vi "BROOKFIELD_EXT-MODE_STATE.vi"() -> ()   [LabVIEW 2019]
uses:
  Brookfield_type-def.ctl
  <vilib>/Instr/_visa.llb/VISA Configure Serial Port (Instr).vi
panel:
  out "error out":errorcluster
  in  "Conductivity Port":refnum<visa-resource-name>="COM5"
  in  "Read Stop":bool
  in  "Disconnect":bool
  out "Enum":T1
  in  "Read Start":bool
  in  "Stop":bool
  in  "Set Speed":bool
  in  "Zero":bool
  out "temp":dbl
  out "torque%":dbl
  out "Control Circuitry Enabled":bool
  out "Motor On":bool
  out "Motor Stopped":bool
  out "Auto-zero Complete":bool
  out "Motor Circuit Error":bool
  out "Diagnostics Error":bool
  out "Invalid Command Received":bool
  out "Torque% Offset":dbl
  in  "rpm setpoint":i32=60
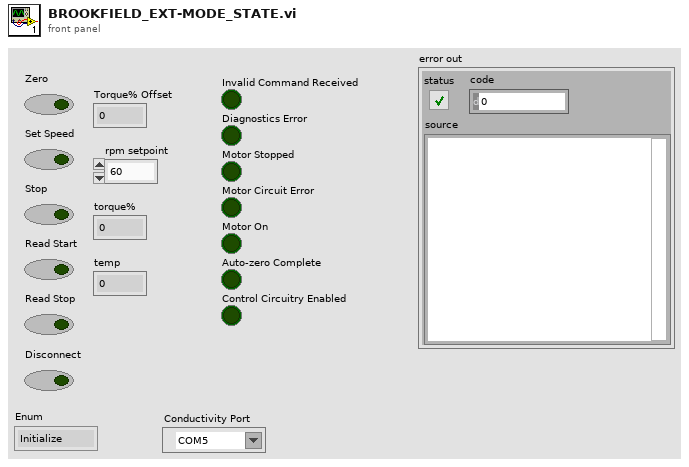
[diagram p1: front panel]
types:
  T1 = typedef "Brookfield_type-def.ctl" = enum16{"Initialize", "Enable", "Ready", "Zero", "Set Speed", "Read", "Stop Motor", "Error", "Disconnect"}
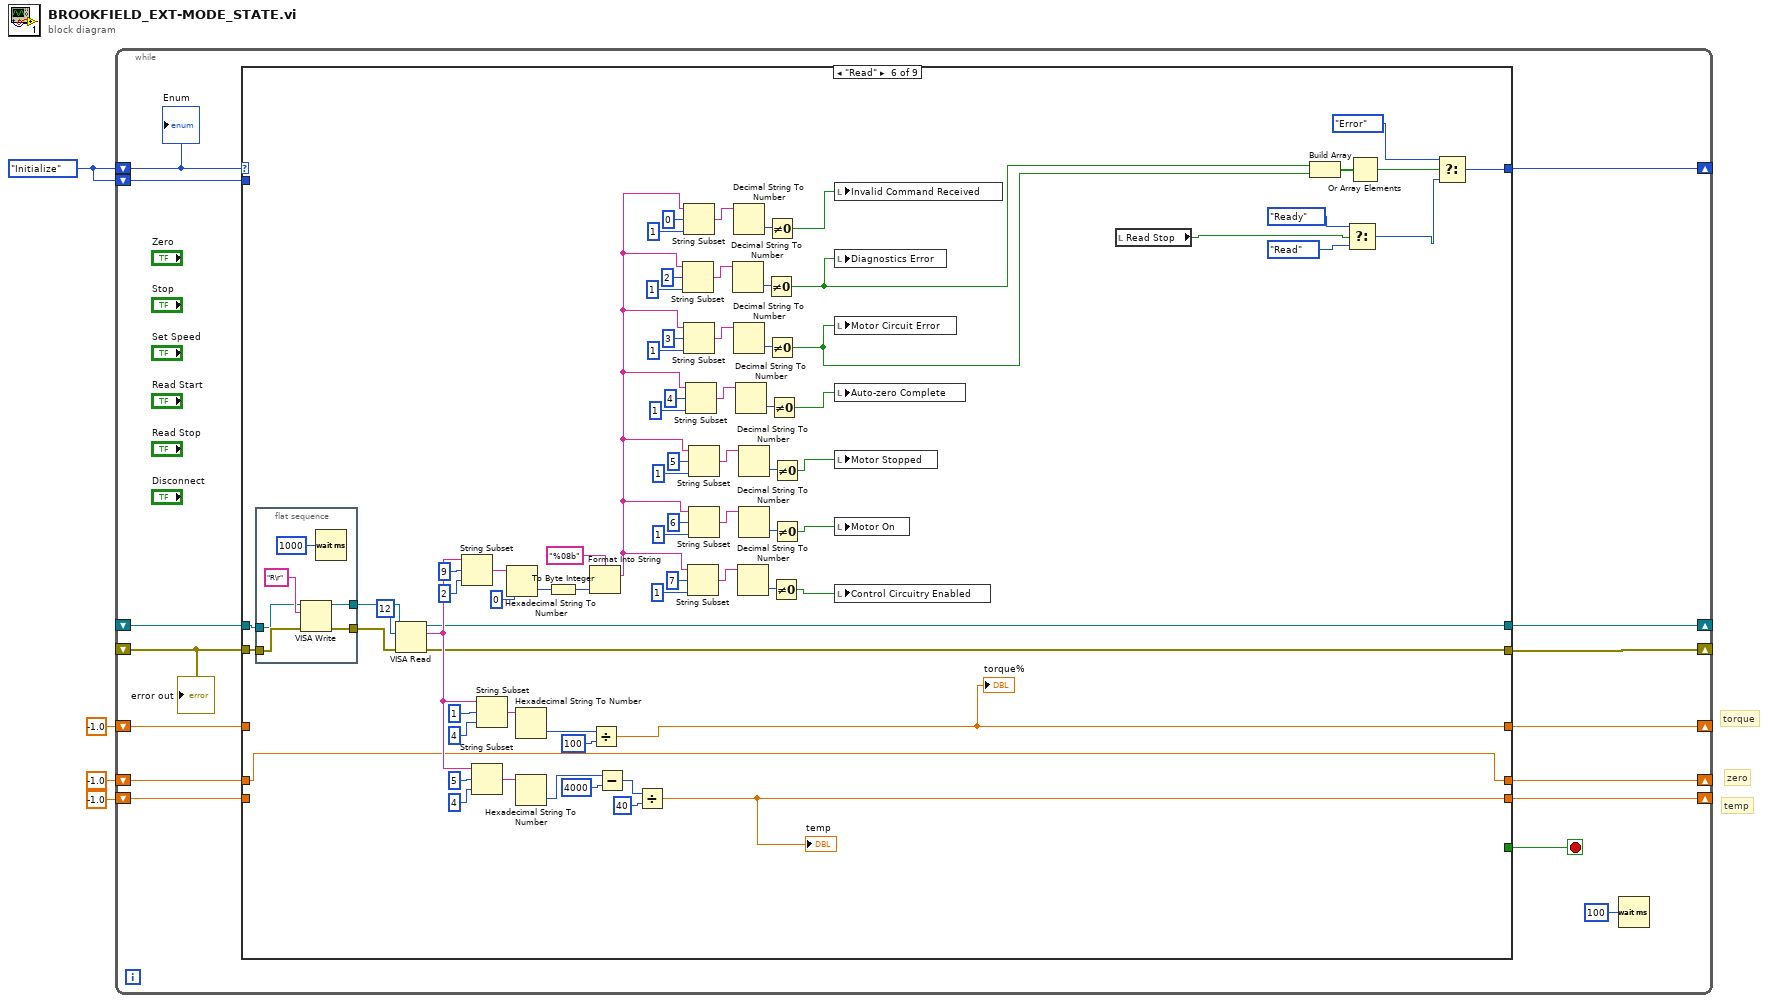
[diagram p0: block diagram]
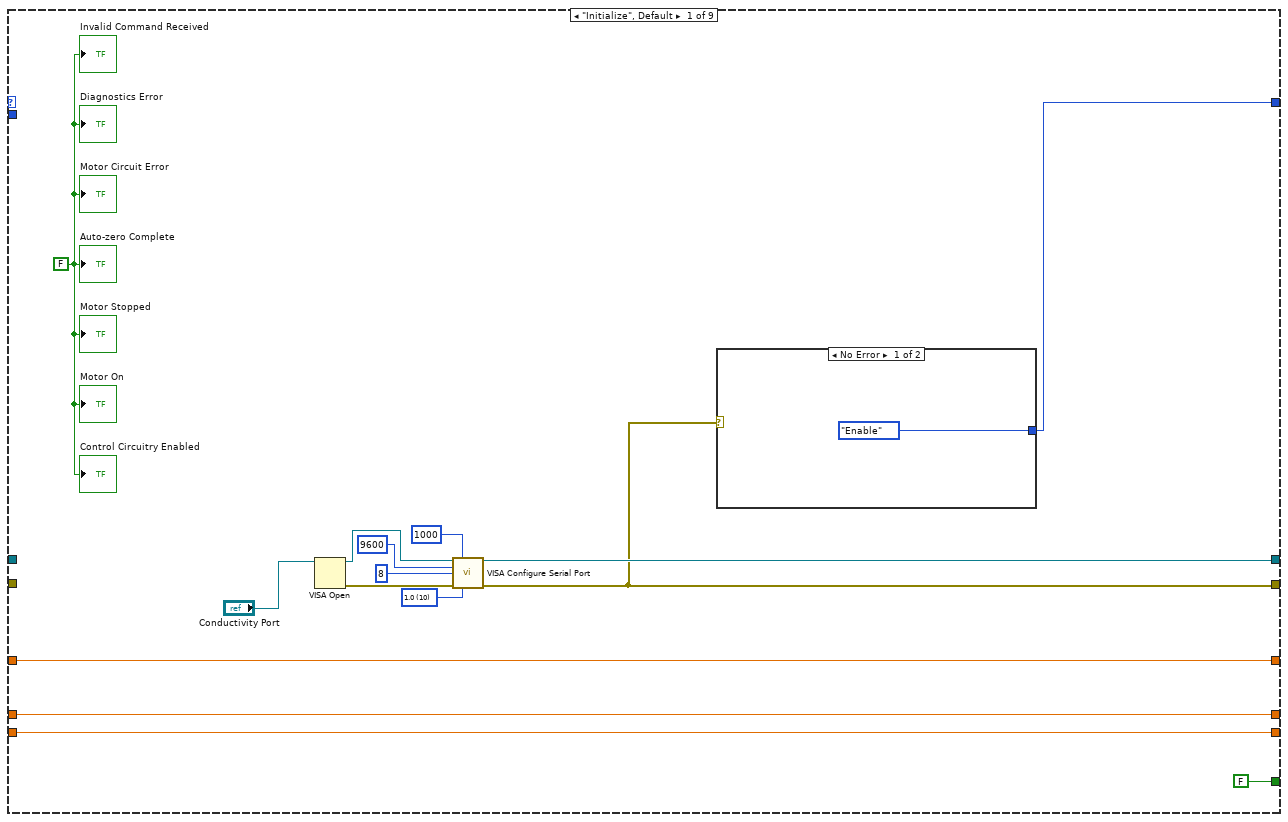
[diagram p2: hidden frame]
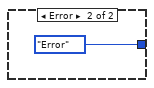
[diagram p3: hidden frame]
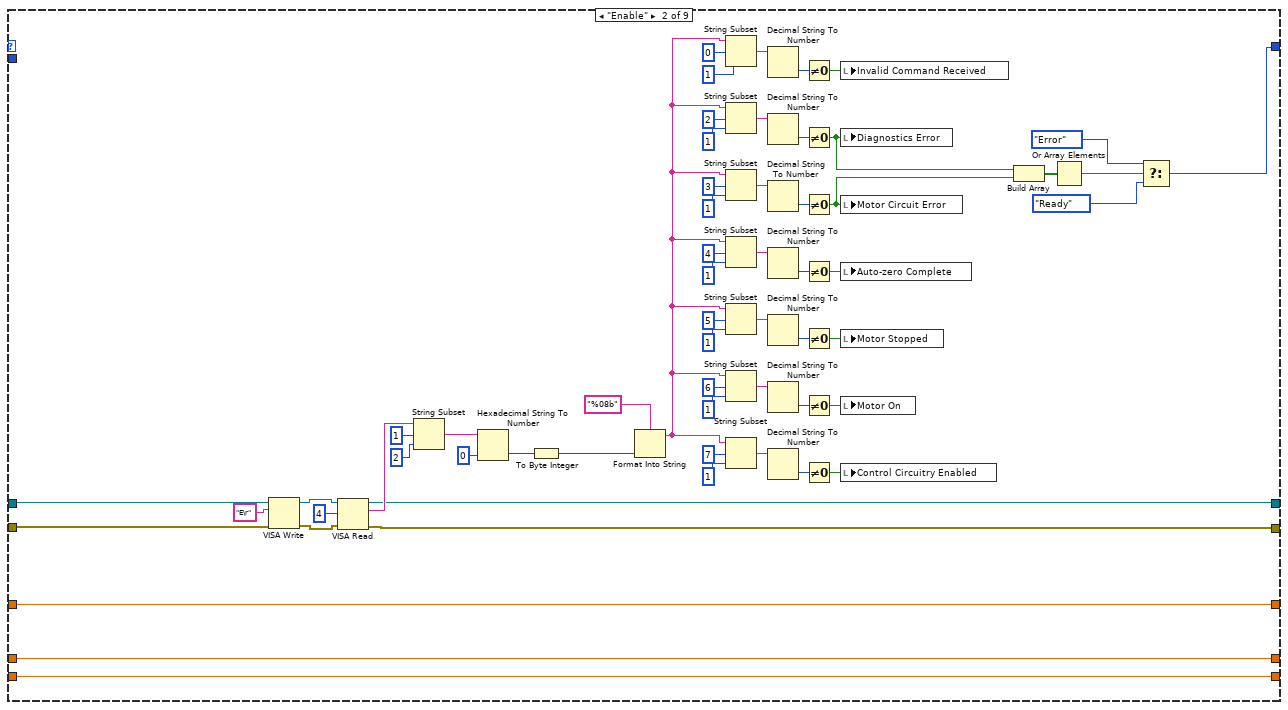
[diagram p4: hidden frame]
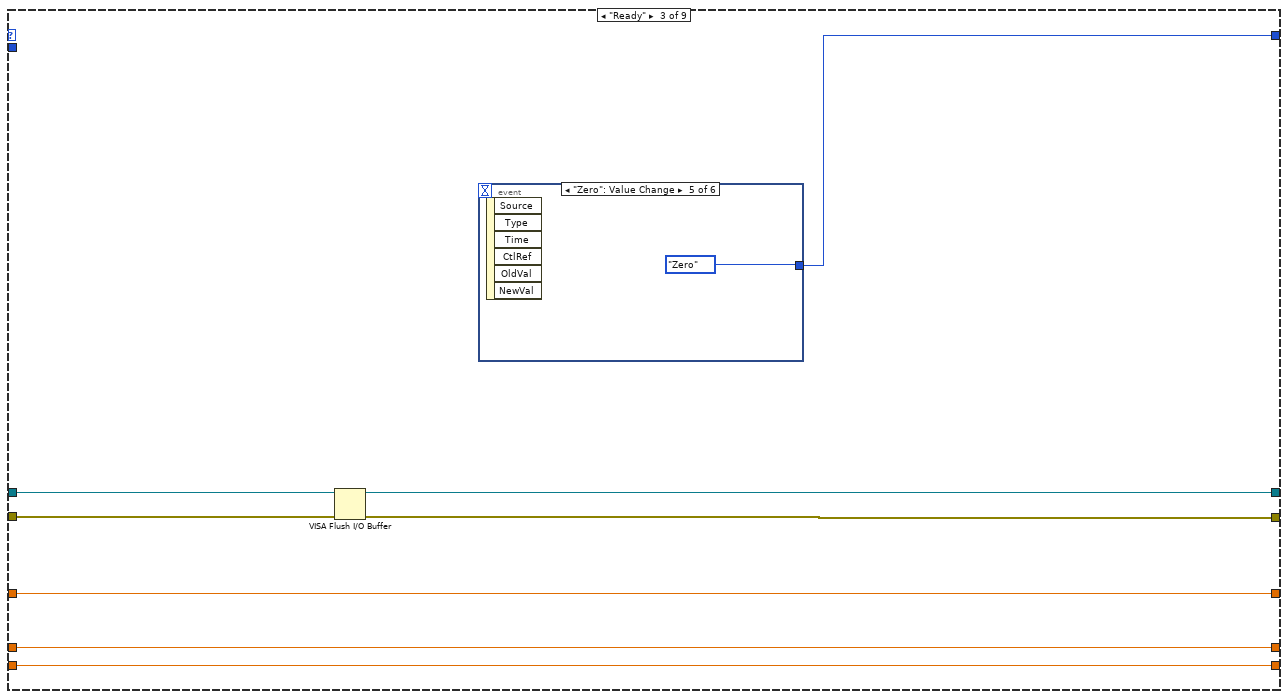
[diagram p5: hidden frame]
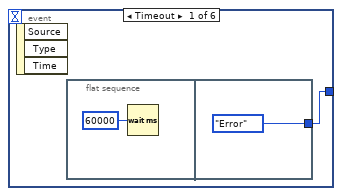
[diagram p6: hidden frame]
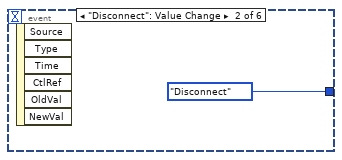
[diagram p7: hidden frame]
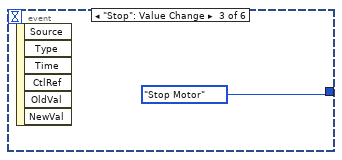
[diagram p8: hidden frame]
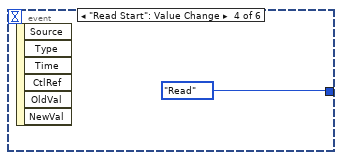
[diagram p9: hidden frame]
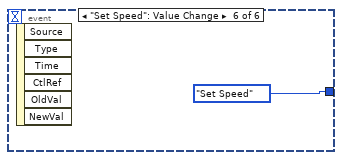
[diagram p10: hidden frame]
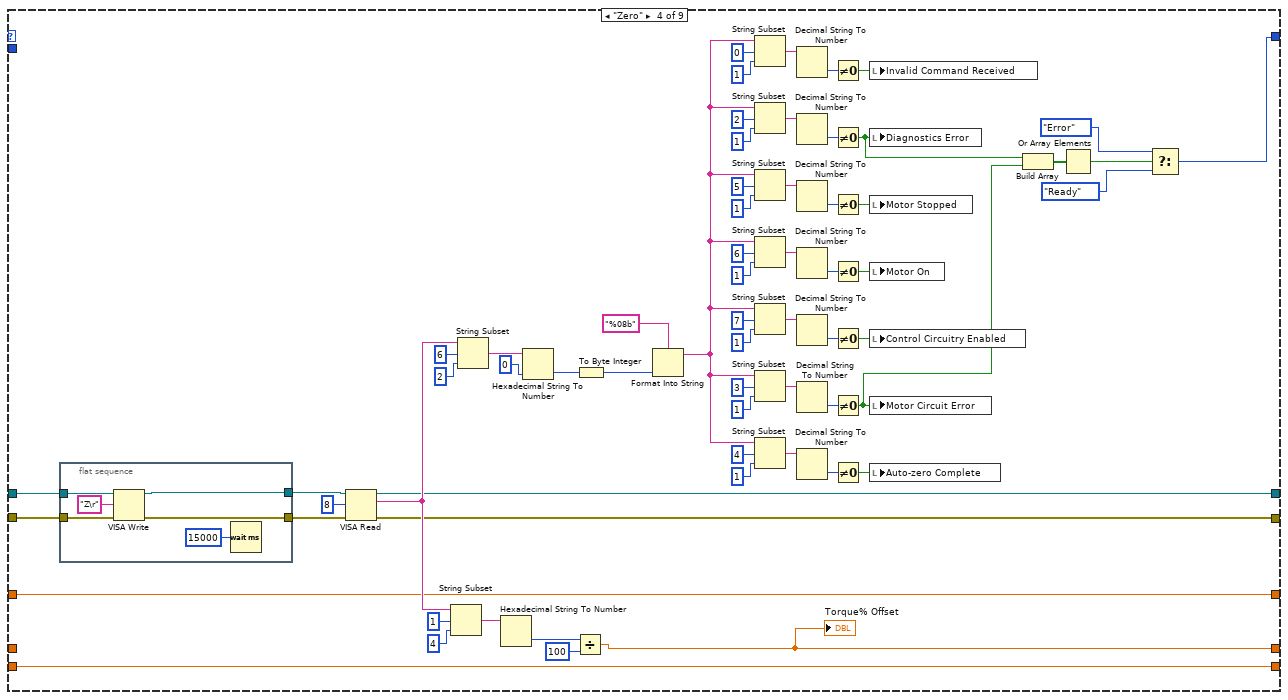
[diagram p11: hidden frame]
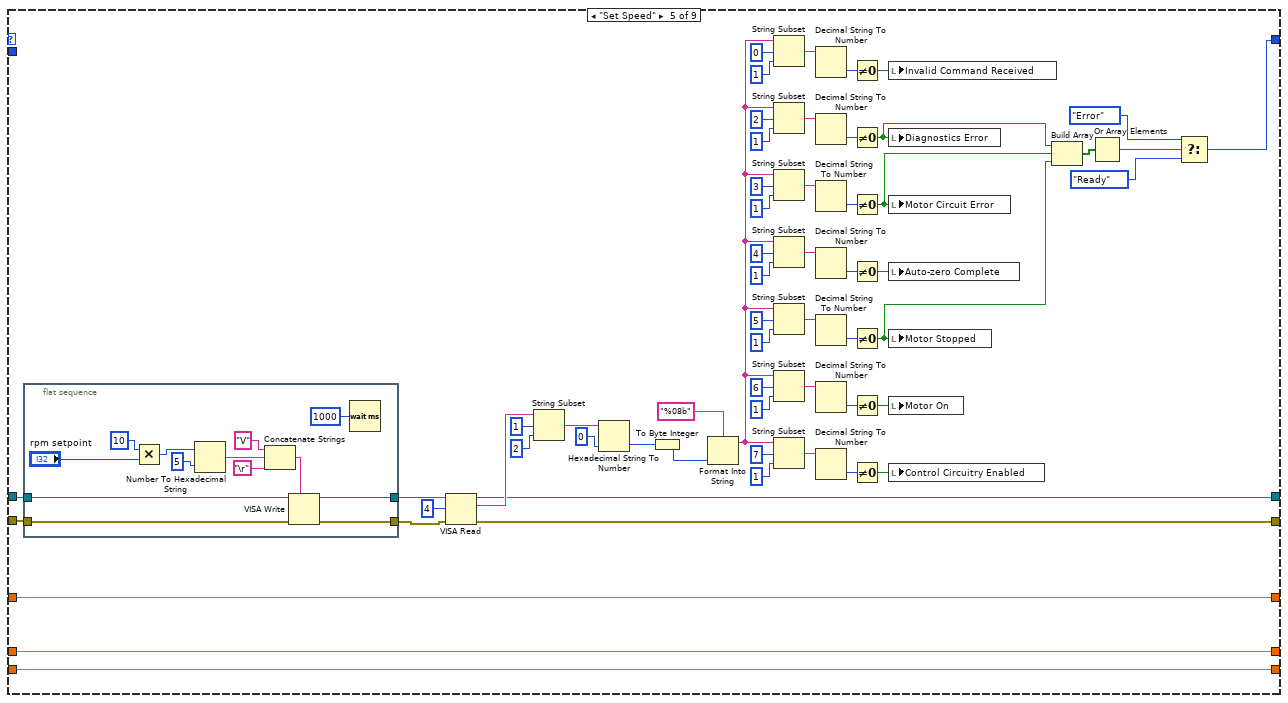
[diagram p12: hidden frame]
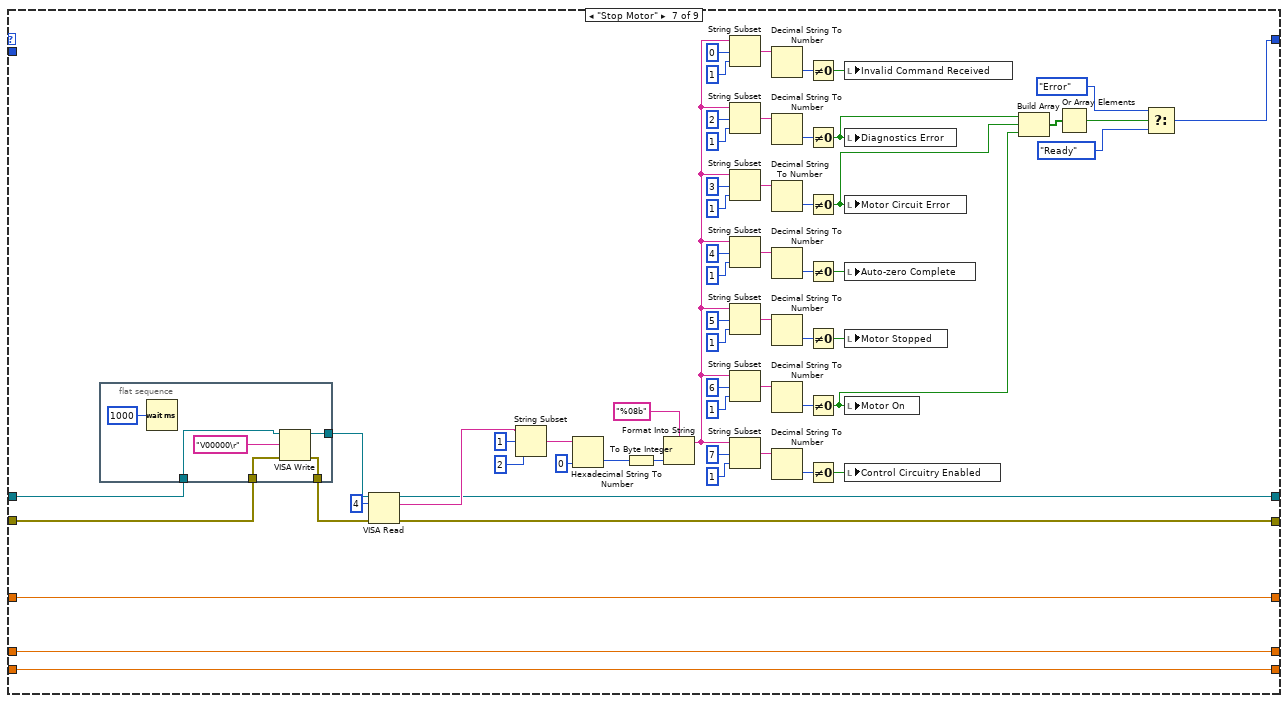
[diagram p13: hidden frame]
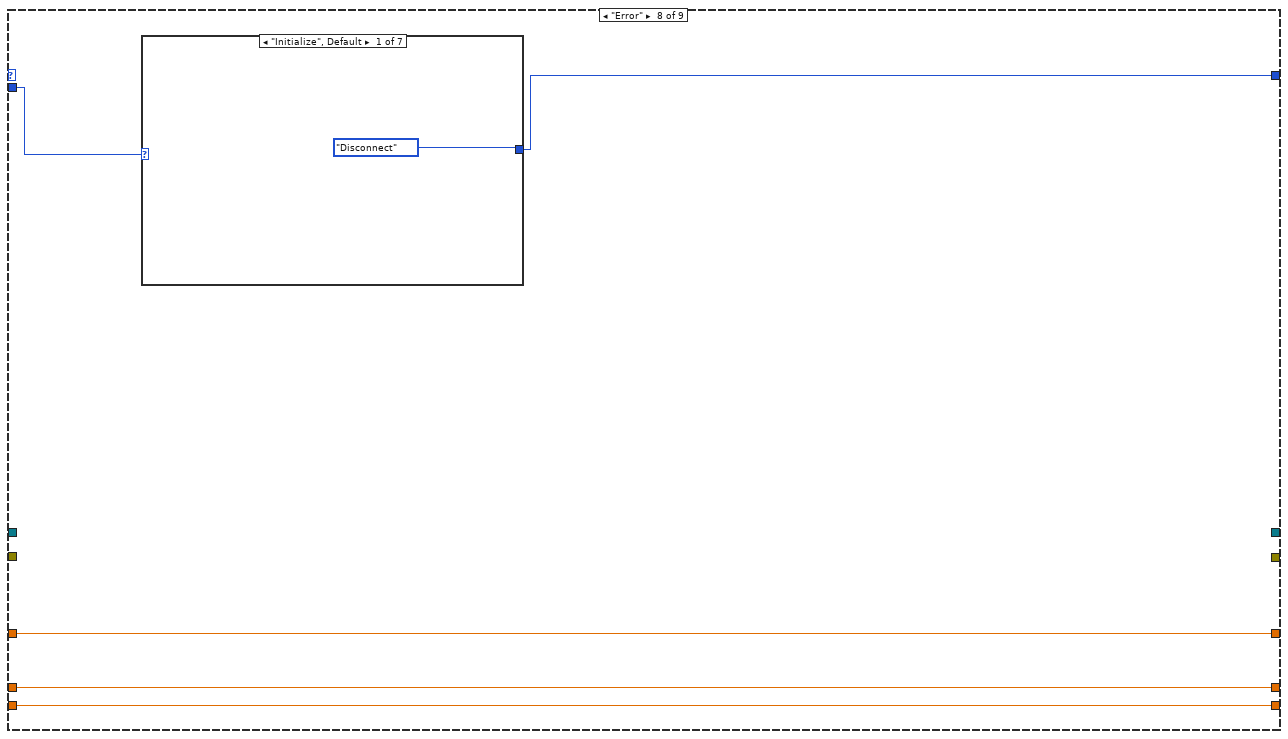
[diagram p14: hidden frame]
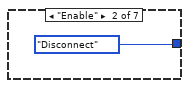
[diagram p15: hidden frame]
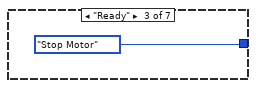
[diagram p16: hidden frame]
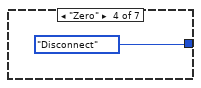
[diagram p17: hidden frame]
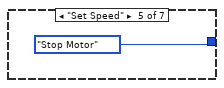
[diagram p18: hidden frame]
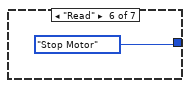
[diagram p19: hidden frame]
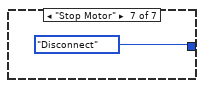
[diagram p20: hidden frame]
diagram:
  w4 = Brookfield_type-def."Initialize"
  # "temp"
  # "zero"
  # "torque"
  n1 = while {
    shift-right: [w13] -> _
    shift-left: w4 -> [w19]
    shift-right: [w18] -> _
    shift-left: _ -> [w16]
    shift-right: [w17] -> _
    shift-left: _ -> [w15]
    shift-right: [w8] -> _
    shift-left: -1.0 -> [w11]
    shift-right: [w9] -> _
    shift-left: -1.0 -> [w6]
    shift-left: w4 -> [w12]
    shift-right: [w7] -> _
    shift-left: -1.0 -> [w10]
    stop <- w14 stop-if-true
    n2 = case shown="\"Read\"" w19 {
      tunnel: [w26 w47 w98 w123 w199 w273 w350 _ _] -> w18
      tunnel: [w25 w48 w97 w124 w200 w272 w351 _ _] -> w17
      tunnel: w16 -> [_ w95 w99 w126 w185 w261 w337 _ w417]
      tunnel: w15 -> [_ w94 w100 w125 w186 w262 w338 _ w416]
      tunnel: [FALSE _ _ _ _ _ _ _ w415] -> w14
      tunnel: [w23 w40 w104 w116 w194 w268 w345 w403 _] -> w13
      tunnel: [w22 w39 w103 w115 w189 w264 w341 w402 w414] -> w8
      tunnel: [w20 w37 w101 w114 w187 w265 w339 w400 w412] -> w9
      tunnel: [w21 w38 w102 w113 w188 w263 w340 w401 w413] -> w7
      tunnel: w12 -> [_ _ _ _ _ _ _ w404 _]
      tunnel: w11 -> [w22 w39 w103 w115 w189 _ w341 w402 w414]
      tunnel: w10 -> [w21 w38 w102 _ w188 w263 w340 w401 w413]
      tunnel: w6 -> [w20 w37 w101 w114 w187 _ w339 w400 w412]
      frame "Initialize", Default {
        w27 = FALSE
        w28 = u16 10 items=["1.0"=10, "1.5"=15, "2.0"=20] ("stop bits (10: 1 bit)")
        n3 = VISA Open(VISA resource name="Conductivity Port") -> (VISA resource name=w34:refnum<visa-resource-name>, error out=w33:errorcluster)  [unwired: 4 in]
        n4 = call-poly "VISA Configure Serial Port"("VISA resource name"=w34, "timeout (10sec)"=u32 1000, "baud rate (9600)"=u32 9600, "data bits (8)"=u16 8, "error in (no error)"=w33, "stop bits (10: 1 bit)"=w28) -> ("VISA resource name out"=w26:refnum<visa-resource-name>, "error out"=w25:errorcluster)  [unwired: 8 in]
        n5 = case shown="No Error" w25 {
          tunnel: [Brookfield_type-def."Enable" Brookfield_type-def."Error"] -> w23
          frame No Error {
          }
          frame Error {
          }
        }
        "Invalid Command Received" <- w27
        "Diagnostics Error" <- w27
        "Motor Circuit Error" <- w27
        "Auto-zero Complete" <- w27
        "Motor Stopped" <- w27
        "Motor On" <- w27
        "Control Circuitry Enabled" <- w27
      }
      frame "Enable" {
        n6 = VISA Write(VISA resource name=w95, write buffer="E\r", error in (no error)=w94) -> (VISA resource name out=w49:refnum<visa-resource-name>, error out=w50:errorcluster)  [unwired: 1 out]
        n7 = VISA Read(VISA resource name=w49, byte count=u32 4, error in (no error)=w50) -> (VISA resource name out=w47:refnum<visa-resource-name>, read buffer=w93:string, error out=w48:errorcluster)  [unwired: 1 out]
        n8 = String Subset(string=w93, offset (0)=1, length (rest)=2 ("length (rest)")) -> (substring=w87:string)
        n9 = Hexadecimal String To Number(string=w87, default (0uL)=u32 0 ("default (0 U32)")) -> (number=w83:u32)  [unwired: 1 in, 1 out]
        n10 = To Byte Integer(number=w83) -> (8bit integer=w84:i8)
        n11 = Format Into String(format string="%08b", w84) -> (resulting string=w70:string)  [unwired: 2 in, 1 out]
        n12 = String Subset(string=w70, offset (0)=0, length (rest)=1 ("length (rest)")) -> (substring=w86:string)
        n13 = String Subset(string=w70, offset (0)=2, length (rest)=1 ("length (rest)")) -> (substring=w81:string)
        n14 = String Subset(string=w70, offset (0)=3, length (rest)=1 ("length (rest)")) -> (substring=w80:string)
        n15 = String Subset(string=w70, offset (0)=4, length (rest)=1 ("length (rest)")) -> (substring=w77:string)
        n16 = String Subset(string=w70, offset (0)=5, length (rest)=1 ("length (rest)")) -> (substring=w76:string)
        n17 = String Subset(string=w70, offset (0)=6, length (rest)=1 ("length (rest)")) -> (substring=w73:string)
        n18 = String Subset(string=w70, offset (0)=7, length (rest)=1 ("length (rest)")) -> (substring=w72:string)
        n19 = Decimal String To Number(string=w86) -> (number=w85:i32)  [unwired: 2 in, 1 out]
        n20 = Decimal String To Number(string=w81) -> (number=w82:i32)  [unwired: 2 in, 1 out]
        n21 = Decimal String To Number(string=w80) -> (number=w79:i32)  [unwired: 2 in, 1 out]
        n22 = Decimal String To Number(string=w77) -> (number=w78:i32)  [unwired: 2 in, 1 out]
        n23 = Decimal String To Number(string=w76) -> (number=w75:i32)  [unwired: 2 in, 1 out]
        n24 = Decimal String To Number(string=w73) -> (number=w74:i32)  [unwired: 2 in, 1 out]
        n25 = Decimal String To Number(string=w72) -> (number=w71:i32)  [unwired: 2 in, 1 out]
        n26 = Not Equal To 0?(x=w85) -> (x != 0?=w88:bool)
        n27 = Not Equal To 0?(x=w82) -> (x != 0?=w46:bool)
        n28 = Not Equal To 0?(x=w79) -> (x != 0?=w45:bool)
        n29 = Not Equal To 0?(x=w78) -> (x != 0?=w89:bool)
        n30 = Not Equal To 0?(x=w75) -> (x != 0?=w90:bool)
        n31 = Not Equal To 0?(x=w74) -> (x != 0?=w91:bool)
        n32 = Not Equal To 0?(x=w71) -> (x != 0?=w92:bool)
        n33 = local write "Invalid Command Received"(w88) -> ()
        n34 = local write "Diagnostics Error"(w46) -> ()
        n35 = local write "Motor Circuit Error"(w45) -> ()
        n36 = local write "Auto-zero Complete"(w89) -> ()
        n37 = local write "Motor Stopped"(w90) -> ()
        n38 = local write "Motor On"(w91) -> ()
        n39 = local write "Control Circuitry Enabled"(w92) -> ()
        n40 = Build Array(w46, w45) -> (w44:bool[])
        n41 = Or Array Elements(Boolean array=w44) -> (logical OR=w43:bool)
        n42 = Select(t=Brookfield_type-def."Error", s=w43, f=Brookfield_type-def."Ready") -> (s? t:f=w40:T1)
      }
      frame "Ready" {
        n43 = VISA Flush I/O Buffer(VISA resource name=w99, error in (no error)=w100) -> (VISA resource name out=w98:refnum<visa-resource-name>, error out=w97:errorcluster)  [unwired: 1 in]
        n44 = event shown="[4] \"Zero\": Value Change" {
          selector: _ -> [_ _ _ _ _ _]
          dyn-events: _ -> [_ _ _ _ _ _]
          timeout: _ -> [_ _ _ _ _ _]
          tunnel: [w105 Brookfield_type-def."Disconnect" Brookfield_type-def."Stop Motor" Brookfield_type-def."Read" Brookfield_type-def."Zero" Brookfield_type-def."Set Speed"] -> w104
          event Timeout {
            n45 = event-data() -> ()  [unwired: 1 in, 3 out]
            n46 = flat-sequence {
              tunnel: [Brookfield_type-def."Error"] -> w105
              frame #0 {
                n47 = Wait (ms)(milliseconds to wait=u32 60000) -> ()  [unwired: 1 out]
              }
              frame #1 {
              }
            }
          }
          event "Disconnect": Value Change {
            n48 = event-data() -> ()  [unwired: 1 in, 6 out]
          }
          event "Stop": Value Change {
            n49 = event-data() -> ()  [unwired: 1 in, 6 out]
          }
          event "Read Start": Value Change {
            n50 = event-data() -> ()  [unwired: 1 in, 6 out]
          }
          event "Zero": Value Change {
            n51 = event-data() -> ()  [unwired: 1 in, 6 out]
          }
          event "Set Speed": Value Change {
            n52 = event-data() -> ()  [unwired: 1 in, 6 out]
          }
        }
      }
      frame "Zero" {
        n53 = flat-sequence {
          tunnel: [w182] -> w150
          tunnel: [w181] -> w149
          tunnel: w126 -> [w179]
          tunnel: w125 -> [w178]
          frame #0 {
            n54 = VISA Write(VISA resource name=w179, write buffer="Z\r", error in (no error)=w178) -> (VISA resource name out=w181:refnum<visa-resource-name>, error out=w182:errorcluster)  [unwired: 1 out]
            n55 = Wait (ms)(milliseconds to wait=u32 15000) -> ()  [unwired: 1 out]
          }
        }
        n56 = VISA Read(VISA resource name=w149, byte count=u32 8, error in (no error)=w150) -> (VISA resource name out=w123:refnum<visa-resource-name>, read buffer=w171:string, error out=w124:errorcluster)  [unwired: 1 out]
        n57 = String Subset(string=w171, offset (0)=1, length (rest)=4 ("length (rest)")) -> (substring=w151:string)
        n58 = String Subset(string=w171, offset (0)=6, length (rest)=2 ("length (rest)")) -> (substring=w153:string)
        n59 = Hexadecimal String To Number(string=w151) -> (number=w152:u32)  [unwired: 2 in, 1 out]
        n60 = Hexadecimal String To Number(string=w153, default (0uL)=u32 0 ("default (0 U32)")) -> (number=w157:u32)  [unwired: 1 in, 1 out]
        n61 = Divide(x=w152, y=u32 100) -> (x/y=w113:dbl)
        "Torque% Offset" <- w113
        n62 = To Byte Integer(number=w157) -> (8bit integer=w156:i8)
        n63 = Format Into String(format string="%08b", w156) -> (resulting string=w170:string)  [unwired: 2 in, 1 out]
        n64 = String Subset(string=w170, offset (0)=0, length (rest)=1 ("length (rest)")) -> (substring=w154:string)
        n65 = String Subset(string=w170, offset (0)=2, length (rest)=1 ("length (rest)")) -> (substring=w159:string)
        n66 = String Subset(string=w170, offset (0)=5, length (rest)=1 ("length (rest)")) -> (substring=w164:string)
        n67 = String Subset(string=w170, offset (0)=6, length (rest)=1 ("length (rest)")) -> (substring=w167:string)
        n68 = String Subset(string=w170, offset (0)=7, length (rest)=1 ("length (rest)")) -> (substring=w168:string)
        n69 = String Subset(string=w170, offset (0)=3, length (rest)=1 ("length (rest)")) -> (substring=w160:string)
        n70 = String Subset(string=w170, offset (0)=4, length (rest)=1 ("length (rest)")) -> (substring=w163:string)
        n71 = Decimal String To Number(string=w154) -> (number=w155:i32)  [unwired: 2 in, 1 out]
        n72 = Decimal String To Number(string=w159) -> (number=w158:i32)  [unwired: 2 in, 1 out]
        n73 = Decimal String To Number(string=w164) -> (number=w165:i32)  [unwired: 2 in, 1 out]
        n74 = Decimal String To Number(string=w167) -> (number=w166:i32)  [unwired: 2 in, 1 out]
        n75 = Decimal String To Number(string=w168) -> (number=w169:i32)  [unwired: 2 in, 1 out]
        n76 = Decimal String To Number(string=w160) -> (number=w161:i32)  [unwired: 2 in, 1 out]
        n77 = Decimal String To Number(string=w163) -> (number=w162:i32)  [unwired: 2 in, 1 out]
        n78 = Not Equal To 0?(x=w155) -> (x != 0?=w176:bool)
        n79 = Not Equal To 0?(x=w158) -> (x != 0?=w118:bool)
        n80 = Not Equal To 0?(x=w165) -> (x != 0?=w174:bool)
        n81 = Not Equal To 0?(x=w166) -> (x != 0?=w173:bool)
        n82 = Not Equal To 0?(x=w169) -> (x != 0?=w172:bool)
        n83 = Not Equal To 0?(x=w161) -> (x != 0?=w117:bool)
        n84 = Not Equal To 0?(x=w162) -> (x != 0?=w175:bool)
        n85 = local write "Invalid Command Received"(w176) -> ()
        n86 = local write "Diagnostics Error"(w118) -> ()
        n87 = local write "Motor Stopped"(w174) -> ()
        n88 = local write "Motor On"(w173) -> ()
        n89 = local write "Control Circuitry Enabled"(w172) -> ()
        n90 = local write "Motor Circuit Error"(w117) -> ()
        n91 = local write "Auto-zero Complete"(w175) -> ()
        n92 = Build Array(w118, w117) -> (w122:bool[])
        n93 = Or Array Elements(Boolean array=w122) -> (logical OR=w121:bool)
        n94 = Select(t=Brookfield_type-def."Error", s=w121, f=Brookfield_type-def."Ready") -> (s? t:f=w116:T1)
      }
      frame "Set Speed" {
        n95 = flat-sequence {
          tunnel: w186 -> [w245]
          tunnel: w185 -> [w244]
          tunnel: [w243] -> w184
          tunnel: [w242] -> w183
          frame #0 {
            n96 = Multiply(x=10, y="rpm setpoint") -> (x*y=w252:i32)
            n97 = Number To Hexadecimal String(1:i16 5 ("width (-)"), 2:w252) -> (0:w251:string)
            n98 = Concatenate Strings("V" ("string"), w251, "\r") -> (w250:string)
            n99 = VISA Write(VISA resource name=w244, write buffer=w250, error in (no error)=w245) -> (VISA resource name out=w242:refnum<visa-resource-name>, error out=w243:errorcluster)  [unwired: 1 out]
            n100 = Wait (ms)(milliseconds to wait=u32 1000) -> ()  [unwired: 1 out]
          }
        }
        n101 = VISA Read(VISA resource name=w183, byte count=u32 4, error in (no error)=w184) -> (VISA resource name out=w199:refnum<visa-resource-name>, read buffer=w241:string, error out=w200:errorcluster)  [unwired: 1 out]
        n102 = String Subset(string=w241, offset (0)=1, length (rest)=2 ("length (rest)")) -> (substring=w237:string)
        n103 = Hexadecimal String To Number(string=w237, default (0uL)=u32 0 ("default (0 U32)")) -> (number=w233:u32)  [unwired: 1 in, 1 out]
        n104 = To Byte Integer(number=w233) -> (8bit integer=w234:i8)
        n105 = Format Into String(format string="%08b", w234) -> (resulting string=w220:string)  [unwired: 2 in, 1 out]
        n106 = String Subset(string=w220, offset (0)=0, length (rest)=1 ("length (rest)")) -> (substring=w236:string)
        n107 = String Subset(string=w220, offset (0)=2, length (rest)=1 ("length (rest)")) -> (substring=w231:string)
        n108 = String Subset(string=w220, offset (0)=3, length (rest)=1 ("length (rest)")) -> (substring=w230:string)
        n109 = String Subset(string=w220, offset (0)=4, length (rest)=1 ("length (rest)")) -> (substring=w227:string)
        n110 = String Subset(string=w220, offset (0)=5, length (rest)=1 ("length (rest)")) -> (substring=w226:string)
        n111 = String Subset(string=w220, offset (0)=6, length (rest)=1 ("length (rest)")) -> (substring=w223:string)
        n112 = String Subset(string=w220, offset (0)=7, length (rest)=1 ("length (rest)")) -> (substring=w222:string)
        n113 = Decimal String To Number(string=w236) -> (number=w235:i32)  [unwired: 2 in, 1 out]
        n114 = Decimal String To Number(string=w231) -> (number=w232:i32)  [unwired: 2 in, 1 out]
        n115 = Decimal String To Number(string=w230) -> (number=w229:i32)  [unwired: 2 in, 1 out]
        n116 = Decimal String To Number(string=w227) -> (number=w228:i32)  [unwired: 2 in, 1 out]
        n117 = Decimal String To Number(string=w226) -> (number=w225:i32)  [unwired: 2 in, 1 out]
        n118 = Decimal String To Number(string=w223) -> (number=w224:i32)  [unwired: 2 in, 1 out]
        n119 = Decimal String To Number(string=w222) -> (number=w221:i32)  [unwired: 2 in, 1 out]
        n120 = Not Equal To 0?(x=w235) -> (x != 0?=w238:bool)
        n121 = Not Equal To 0?(x=w232) -> (x != 0?=w192:bool)
        n122 = Not Equal To 0?(x=w229) -> (x != 0?=w193:bool)
        n123 = Not Equal To 0?(x=w228) -> (x != 0?=w239:bool)
        n124 = Not Equal To 0?(x=w225) -> (x != 0?=w190:bool)
        n125 = Not Equal To 0?(x=w224) -> (x != 0?=w191:bool)
        n126 = Not Equal To 0?(x=w221) -> (x != 0?=w240:bool)
        n127 = local write "Invalid Command Received"(w238) -> ()
        n128 = local write "Diagnostics Error"(w192) -> ()
        n129 = local write "Motor Circuit Error"(w193) -> ()
        n130 = local write "Auto-zero Complete"(w239) -> ()
        n131 = local write "Motor Stopped"(w190) -> ()
        n132 = local write "Motor On"(w191) -> ()
        n133 = local write "Control Circuitry Enabled"(w240) -> ()
        n134 = Build Array(w192, w193, w190) -> (w198:bool[])
        n135 = Or Array Elements(Boolean array=w198) -> (logical OR=w197:bool)
        n136 = Select(t=Brookfield_type-def."Error", s=w197, f=Brookfield_type-def."Ready") -> (s? t:f=w194:T1)
      }
      frame "Read" {
        n137 = flat-sequence {
          tunnel: w262 -> [w333]
          tunnel: w261 -> [w331]
          tunnel: [w330] -> w260
          tunnel: [w329] -> w259
          frame #0 {
            n138 = VISA Write(VISA resource name=w331, write buffer="R\r", error in (no error)=w333) -> (VISA resource name out=w329:refnum<visa-resource-name>, error out=w330:errorcluster)  [unwired: 1 out]
            n139 = Wait (ms)(milliseconds to wait=u32 1000) -> ()  [unwired: 1 out]
          }
        }
        n140 = VISA Read(VISA resource name=w259, byte count=u32 12, error in (no error)=w260) -> (VISA resource name out=w273:refnum<visa-resource-name>, read buffer=w313:string, error out=w272:errorcluster)  [unwired: 1 out]
        n141 = String Subset(string=w313, offset (0)=9, length (rest)=2 ("length (rest)")) -> (substring=w312:string)
        n142 = String Subset(string=w313, offset (0)=5, length (rest)=4 ("length (rest)")) -> (substring=w319:string)
        n143 = String Subset(string=w313, offset (0)=1, length (rest)=4 ("length (rest)")) -> (substring=w325:string)
        n144 = Hexadecimal String To Number(string=w312, default (0uL)=u32 0 ("default (0 U32)")) -> (number=w304:u32)  [unwired: 1 in, 1 out]
        n145 = Hexadecimal String To Number(string=w325) -> (number=w324:u32)  [unwired: 2 in, 1 out]
        n146 = Hexadecimal String To Number(string=w319) -> (number=w318:u32)  [unwired: 2 in, 1 out]
        n147 = To Byte Integer(number=w304) -> (8bit integer=w305:i8)
        n148 = Format Into String(format string="%08b", w305) -> (resulting string=w279:string)  [unwired: 2 in, 1 out]
        n149 = Divide(x=w324, y=u32 100) -> (x/y=w264:dbl)
        "torque%" <- w264
        n150 = Subtract(x=w318, y=u32 4000) -> (x-y=w316:u32)
        n151 = Divide(x=w316, y=u32 40) -> (x/y=w265:dbl)
        "temp" <- w265
        n152 = String Subset(string=w279, offset (0)=2, length (rest)=1 ("length (rest)")) -> (substring=w302:string)
        n153 = String Subset(string=w279, offset (0)=0, length (rest)=1 ("length (rest)")) -> (substring=w308:string)
        n154 = String Subset(string=w279, offset (0)=3, length (rest)=1 ("length (rest)")) -> (substring=w297:string)
        n155 = String Subset(string=w279, offset (0)=4, length (rest)=1 ("length (rest)")) -> (substring=w294:string)
        n156 = String Subset(string=w279, offset (0)=7, length (rest)=1 ("length (rest)")) -> (substring=w281:string)
        n157 = String Subset(string=w279, offset (0)=5, length (rest)=1 ("length (rest)")) -> (substring=w289:string)
        n158 = String Subset(string=w279, offset (0)=6, length (rest)=1 ("length (rest)")) -> (substring=w286:string)
        n159 = Decimal String To Number(string=w302) -> (number=w303:i32)  [unwired: 2 in, 1 out]
        n160 = Decimal String To Number(string=w308) -> (number=w307:i32)  [unwired: 2 in, 1 out]
        n161 = Decimal String To Number(string=w297) -> (number=w296:i32)  [unwired: 2 in, 1 out]
        n162 = Decimal String To Number(string=w294) -> (number=w295:i32)  [unwired: 2 in, 1 out]
        n163 = Decimal String To Number(string=w281) -> (number=w280:i32)  [unwired: 2 in, 1 out]
        n164 = Decimal String To Number(string=w289) -> (number=w288:i32)  [unwired: 2 in, 1 out]
        n165 = Decimal String To Number(string=w286) -> (number=w287:i32)  [unwired: 2 in, 1 out]
        n166 = Not Equal To 0?(x=w303) -> (x != 0?=w267:bool)
        n167 = Not Equal To 0?(x=w307) -> (x != 0?=w274:bool)
        n168 = Not Equal To 0?(x=w296) -> (x != 0?=w266:bool)
        n169 = Not Equal To 0?(x=w295) -> (x != 0?=w275:bool)
        n170 = Not Equal To 0?(x=w280) -> (x != 0?=w278:bool)
        n171 = Not Equal To 0?(x=w288) -> (x != 0?=w276:bool)
        n172 = Not Equal To 0?(x=w287) -> (x != 0?=w277:bool)
        n173 = local write "Invalid Command Received"(w274) -> ()
        n174 = local write "Diagnostics Error"(w267) -> ()
        n175 = local write "Motor Circuit Error"(w266) -> ()
        n176 = local write "Auto-zero Complete"(w275) -> ()
        n177 = local write "Motor Stopped"(w276) -> ()
        n178 = local write "Motor On"(w277) -> ()
        n179 = local write "Control Circuitry Enabled"(w278) -> ()
        n180 = local read "Read Stop"() -> (w255:bool)
        n181 = Build Array(w267, w266) -> (w269:bool[])
        n182 = Select(t=Brookfield_type-def."Ready", s=w255, f=Brookfield_type-def."Read") -> (s? t:f=w258:T1)
        n183 = Or Array Elements(Boolean array=w269) -> (logical OR=w271:bool)
        n184 = Select(t=Brookfield_type-def."Error", s=w271, f=w258) -> (s? t:f=w268:T1)
      }
      frame "Stop Motor" {
        n185 = flat-sequence {
          tunnel: w338 -> [w398]
          tunnel: w337 -> [w396]
          tunnel: [w395] -> w336
          tunnel: [w394] -> w335
          frame #0 {
            n186 = Wait (ms)(milliseconds to wait=u32 1000) -> ()  [unwired: 1 out]
            n187 = VISA Write(VISA resource name=w396, write buffer="V00000\r", error in (no error)=w398) -> (VISA resource name out=w394:refnum<visa-resource-name>, error out=w395:errorcluster)  [unwired: 1 out]
          }
        }
        n188 = VISA Read(VISA resource name=w335, byte count=u32 4, error in (no error)=w336) -> (VISA resource name out=w350:refnum<visa-resource-name>, read buffer=w371:string, error out=w351:errorcluster)  [unwired: 1 out]
        n189 = String Subset(string=w371, offset (0)=1, length (rest)=2 ("length (rest)")) -> (substring=w376:string)
        n190 = Hexadecimal String To Number(string=w376, default (0uL)=u32 0 ("default (0 U32)")) -> (number=w380:u32)  [unwired: 1 in, 1 out]
        n191 = To Byte Integer(number=w380) -> (8bit integer=w379:i8)
        n192 = Format Into String(format string="%08b", w379) -> (resulting string=w393:string)  [unwired: 2 in, 1 out]
        n193 = String Subset(string=w393, offset (0)=0, length (rest)=1 ("length (rest)")) -> (substring=w377:string)
        n194 = String Subset(string=w393, offset (0)=2, length (rest)=1 ("length (rest)")) -> (substring=w382:string)
        n195 = String Subset(string=w393, offset (0)=3, length (rest)=1 ("length (rest)")) -> (substring=w383:string)
        n196 = String Subset(string=w393, offset (0)=4, length (rest)=1 ("length (rest)")) -> (substring=w386:string)
        n197 = String Subset(string=w393, offset (0)=5, length (rest)=1 ("length (rest)")) -> (substring=w387:string)
        n198 = String Subset(string=w393, offset (0)=6, length (rest)=1 ("length (rest)")) -> (substring=w390:string)
        n199 = String Subset(string=w393, offset (0)=7, length (rest)=1 ("length (rest)")) -> (substring=w391:string)
        n200 = Decimal String To Number(string=w377) -> (number=w378:i32)  [unwired: 2 in, 1 out]
        n201 = Decimal String To Number(string=w382) -> (number=w381:i32)  [unwired: 2 in, 1 out]
        n202 = Decimal String To Number(string=w383) -> (number=w384:i32)  [unwired: 2 in, 1 out]
        n203 = Decimal String To Number(string=w386) -> (number=w385:i32)  [unwired: 2 in, 1 out]
        n204 = Decimal String To Number(string=w387) -> (number=w388:i32)  [unwired: 2 in, 1 out]
        n205 = Decimal String To Number(string=w390) -> (number=w389:i32)  [unwired: 2 in, 1 out]
        n206 = Decimal String To Number(string=w391) -> (number=w392:i32)  [unwired: 2 in, 1 out]
        n207 = Not Equal To 0?(x=w378) -> (x != 0?=w375:bool)
        n208 = Not Equal To 0?(x=w381) -> (x != 0?=w344:bool)
        n209 = Not Equal To 0?(x=w384) -> (x != 0?=w343:bool)
        n210 = Not Equal To 0?(x=w385) -> (x != 0?=w374:bool)
        n211 = Not Equal To 0?(x=w388) -> (x != 0?=w373:bool)
        n212 = Not Equal To 0?(x=w389) -> (x != 0?=w342:bool)
        n213 = Not Equal To 0?(x=w392) -> (x != 0?=w372:bool)
        n214 = local write "Invalid Command Received"(w375) -> ()
        n215 = local write "Diagnostics Error"(w344) -> ()
        n216 = local write "Motor Circuit Error"(w343) -> ()
        n217 = local write "Auto-zero Complete"(w374) -> ()
        n218 = local write "Motor Stopped"(w373) -> ()
        n219 = local write "Motor On"(w342) -> ()
        n220 = local write "Control Circuitry Enabled"(w372) -> ()
        n221 = Build Array(w344, w343, w342) -> (w349:bool[])
        n222 = Or Array Elements(Boolean array=w349) -> (logical OR=w348:bool)
        n223 = Select(t=Brookfield_type-def."Error", s=w348, f=Brookfield_type-def."Ready") -> (s? t:f=w345:T1)
      }
      frame "Error" {
        n224 = case shown="\"Initialize\", Default" w404 {
          tunnel: [Brookfield_type-def."Disconnect" Brookfield_type-def."Disconnect" Brookfield_type-def."Stop Motor" Brookfield_type-def."Disconnect" Brookfield_type-def."Stop Motor" Brookfield_type-def."Stop Motor" Brookfield_type-def."Disconnect"] -> w403
          frame "Initialize", Default {
          }
          frame "Enable" {
          }
          frame "Ready" {
          }
          frame "Zero" {
          }
          frame "Set Speed" {
          }
          frame "Read" {
          }
          frame "Stop Motor" {
          }
        }
      }
      frame "Disconnect" {
        n225 = flat-sequence {
          tunnel: w417 -> [w419]
          tunnel: w416 -> [w418]
          tunnel: [TRUE] -> w415
          frame #0 {
            n226 = VISA Close(VISA resource name=w419, error in (no error)=w418) -> ()  [unwired: 1 out]
          }
          frame #1 {
          }
        }
      }
    }
    n227 = Wait (ms)(milliseconds to wait=u32 100) -> ()  [unwired: 1 out]
    "Enum" <- w19
    "error out" <- w15
  }
